vi "Page_Source_Can_Add_to_Top.vi"(6 "Project Refnum":refnum<vi>, 8 "error in (no error)":errorcluster, 10 "AB_Source in":refnum<class "AB_Source.lvclass">, 11 "AB_Application in":refnum<class "AB_Application.lvclass">) -> (0 "error out":errorcluster, 1 "message":string, 2 "canAddToTop":bool, 3 "AB_Application out":refnum<class "AB_Application.lvclass">)   [LabVIEW 2020, in "AB_Application.lvclass"]
uses:
  <vilib>/AppBuilder/AB_Classes/Application/AB_Application.lvclass
  <vilib>/AppBuilder/AB_Classes/Source/AB_Source.lvclass
  <resource>/Framework/Providers/Common/provcom_StringGlobals.vi
  <vilib>/AppBuilder/AB_Classes/TargetFile/AB_Targetfile.lvclass
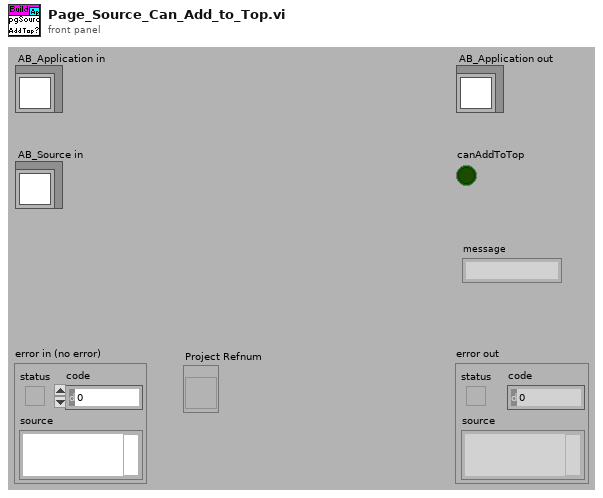
[diagram p1: front panel]
types:
  T1 = typedef "AB_Source.ctl" = cluster{"path":path, "itemID":string, "parentIndex":i32, "sourceInclusion":T2, "destinationIndex":i32, "properties":T3[], "newName":string, "lvfile":bool, "valid":bool, "eng_inBuild":bool, "eng_isNonVILink":bool, "Amalgamation":bool, "Amalgamation Piece":bool, "eng_delimitedName":string, "preventRename":bool}
  T2 = typedef "AB_Source_Inclusion.ctl" = enum16{"IncludeIfReferenced", "Include", "Exclude", "TopLevel"}
  T3 = typedef "AB_Source_Properties.ctl" = cluster{"sourcePropertyType":T4, "value":variant}
  T4 = typedef "AB_Source_Property_Type.ctl" = enum16{"Remove block diagram", "Remove front panel", "Password", "Window has title bar", "Show menu bar", "Show vertical scroll bar", "Show horizontal scroll bar", "Show toolbar", "Show Abort button", "Show fp when called", "Window behavior", "Allow user to close window", "Window run-time position", "Run when opened", "Allow debugging", "Auto error handling", "Generate guard code", "Use stack variables", "Expression folding", "Integer only", "Inline subVI"}
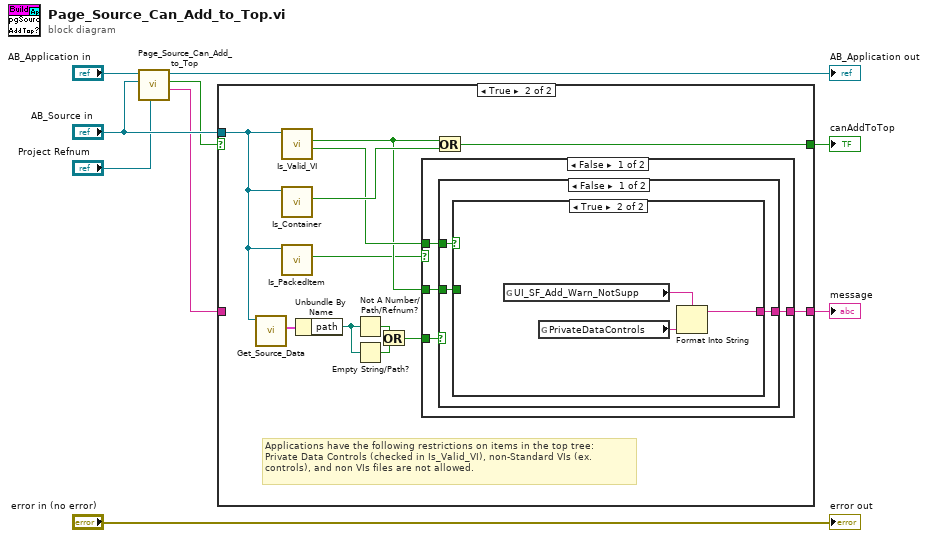
[diagram p0: block diagram]
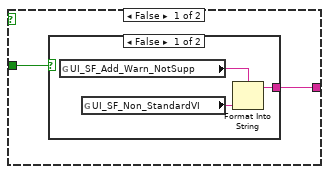
[diagram p3: hidden frame]
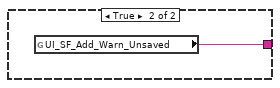
[diagram p5: hidden frame]
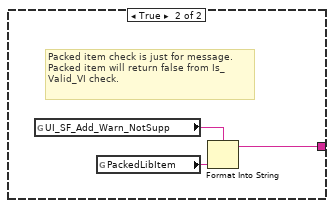
[diagram p6: hidden frame]
diagram:
  n1 = call-parent "Page_Source_Can_Add_to_Top.vi"("Project Refnum"="Project Refnum", "AB_Source in"="AB_Source in", "AB_Targetfile in"="AB_Application in") -> ("message"=w2:string, "canAddToTop"=w3:bool, "AB_Targetfile out"=→"AB_Application out":refnum<class "AB_Application.lvclass">)  [unwired: 5 in, 1 out]
  n2 = case shown="True" w3 {
    selector: w3 -> [w11 _]
    tunnel: [w11 w22] -> w8
    tunnel: [w10 w16] -> w7
    tunnel: "AB_Source in" -> [_ w13]
    tunnel: w2 -> [w10 _]
    frame False {
    }
    frame True {
      # "Applications have the following restrictions on items in the top tree:\nPrivate Data Controls (checked in Is_Valid_VI), non-Standard VIs (ex. controls), and non VIs files are not allowed."
      n3 = call <vilib>:"Get_Source_Data.vi"("Class in"=w13) -> ("data"=w21:T1)  [unwired: 8 in, 2 out]
      n4 = call-dynamic "Is_Valid_VI.vi"("AB_Source in"=w13) -> ("PDC"=w15:bool, "VI"=w14:bool)  [unwired: 7 in, 2 out]
      n5 = call-dynamic "Is_Container.vi"("AB_Source in"=w13) -> ("container"=w23:bool)  [unwired: 8 in, 2 out]
      n6 = call-dynamic "Is_PackedItem.vi"("AB_Source in"=w13) -> ("packed item"=w12:bool)  [unwired: 8 in, 2 out]
      n7 = Unbundle By Name(w21) -> ("path"=w18:path)
      n8 = Not A Number/Path/Refnum?(number/path/refnum=w18) -> (NaN/Path/Refnum?=w19:bool)
      n9 = Empty String/Path?(string/path=w18) -> (empty?=w20:bool)
      n10 = Or(x=w19, y=w20) -> (x .or. y?=w17:bool)
      n11 = case shown="False" w12 {
        tunnel: w17 -> [w27 _]
        tunnel: [w26 w41] -> w16
        tunnel: w15 -> [w25 _]
        tunnel: w14 -> [w24 _]
        frame False {
          n12 = case shown="False" w27 {
            tunnel: w24 -> [w28 _]
            tunnel: w25 -> [w30 _]
            tunnel: [w29 w39] -> w26
            frame False {
              n13 = case shown="True" w30 {
                tunnel: [w32 w36] -> w29
                tunnel: w28 -> [w31 _]
                frame False {
                  n14 = case shown="False" w31 {
                    tunnel: [w33 _] -> w32
                    frame False {
                      n15 = global read "provcom_StringGlobals.vi" "UI_SF_Add_Warn_NotSupp"() -> (w35:string)
                      n16 = global read "provcom_StringGlobals.vi" "UI_SF_Non_StandardVI"() -> (w34:string)
                      n17 = Format Into String(format string=w35, w34) -> (resulting string=w33:string)  [unwired: 2 in, 1 out]
                    }
                    frame True {
                    }
                  }
                }
                frame True {
                  n18 = global read "provcom_StringGlobals.vi" "UI_SF_Add_Warn_NotSupp"() -> (w38:string)
                  n19 = global read "provcom_StringGlobals.vi" "PrivateDataControls"() -> (w37:string)
                  n20 = Format Into String(format string=w38, w37) -> (resulting string=w36:string)  [unwired: 2 in, 1 out]
                }
              }
            }
            frame True {
              n21 = global read "provcom_StringGlobals.vi" "UI_SF_Add_Warn_Unsaved"() -> (w39:string)
            }
          }
        }
        frame True {
          # "Packed item check is just for message. Packed item will return false from Is_Valid_VI check."
          n22 = global read "provcom_StringGlobals.vi" "UI_SF_Add_Warn_NotSupp"() -> (w42:string)
          n23 = global read "provcom_StringGlobals.vi" "PackedLibItem"() -> (w40:string)
          n24 = Format Into String(format string=w42, w40) -> (resulting string=w41:string)  [unwired: 2 in, 1 out]
        }
      }
      n25 = Or(x=w14, y=w23) -> (x .or. y?=w22:bool)
    }
  }
  "canAddToTop" <- w8
  "message" <- w7
  "error out" <- "error in (no error)"
